vi "destroy.vi"(8 "error in":errorcluster, 11 "task token in":refnum<class "cancel token.lvclass">) -> (0 "error out":errorcluster)   [LabVIEW 2013, in "cancel token.lvclass"]
uses:
  cancel token.lvclass
  cancel token.lvclass/cancel token.ctl
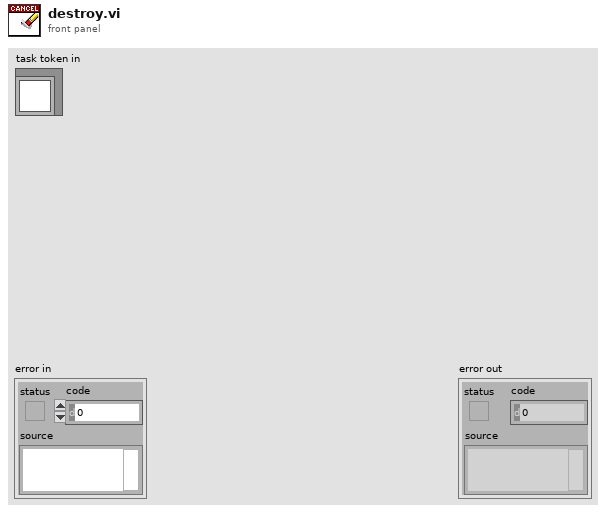
[diagram p1: front panel]
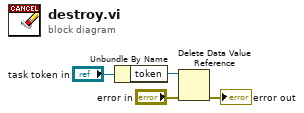
[diagram p0: block diagram]
diagram:
  n1 = Unbundle By Name("task token in") -> ("token"=w1:refnum<data-value>)
  n2 = Delete Data Value Reference(data value reference=w1, error in="error in") -> (error out=→"error out":errorcluster)  [unwired: 1 out]
